vi "swerve_graphing.vi"(10 "wheel offset":dbl format="%_6g", 11 "Pose":dbl[](array[numeric])) -> (2 "Output":cluster{"x out":dbl, "y out":dbl}[](array[cluster]))   [LabVIEW 2020]
uses:
  <vilib>/Analysis/coordinate.llb/2D Cartesian Coordinate Rotation (Scalar).vi
  swerve_globals.vi
  <vilib>/Analysis/NI_AALPro.lvlib
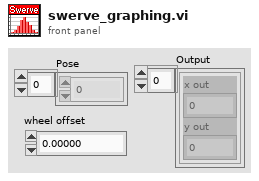
[diagram p1: front panel]
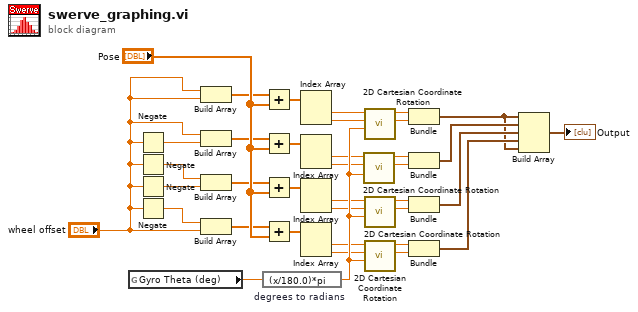
[diagram p0: block diagram]
diagram:
  n1 = global read "swerve_globals.vi" "Gyro Theta (deg)"() -> (w18:dbl)
  n2 = Negate(x="wheel offset") -> (-x=w3:dbl)
  n3 = Negate(x="wheel offset") -> (-x=w1:dbl)
  n4 = Negate(x="wheel offset") -> (-x=w4:dbl)
  n5 = Negate(x="wheel offset") -> (-x=w2:dbl)
  n6 = Build Array("wheel offset", "wheel offset") -> (w24:dbl[])
  n7 = Build Array("wheel offset", w3) -> (w25:dbl[])
  n8 = Build Array(w1, w4) -> (w26:dbl[])
  n9 = Build Array(w2, "wheel offset") -> (w27:dbl[])
  n10 = expression code="(x/180.0)*pi" "degrees to radians"(w18) -> (w23:dbl)
  n11 = Add(x=w24, y="Pose") -> (x+y=w6:dbl[])
  n12 = Add(x=w25, y="Pose") -> (x+y=w7:dbl[])
  n13 = Add(x=w26, y="Pose") -> (x+y=w8:dbl[])
  n14 = Add(x=w27, y="Pose") -> (x+y=w9:dbl[])
  n15 = Index Array(array=w6) -> (element #1=w10:dbl, element #2=w11:dbl)  [unwired: 2 in]
  n16 = Index Array(array=w7) -> (element #1=w12:dbl, element #2=w13:dbl)  [unwired: 2 in]
  n17 = Index Array(array=w8) -> (element #1=w14:dbl, element #2=w15:dbl)  [unwired: 2 in]
  n18 = Index Array(array=w9) -> (element #1=w16:dbl, element #2=w17:dbl)  [unwired: 2 in]
  n19 = call-poly <vilib>:"2D Cartesian Coordinate Rotation.vi"("theta"=w23, "y"=w13, "x"=w12) -> ("y out"=w34:dbl, "x out"=w33:dbl)  [unwired: 6 in, 1 out]
  n20 = call-poly <vilib>:"2D Cartesian Coordinate Rotation.vi"("theta"=w23, "y"=w11, "x"=w10) -> ("y out"=w36:dbl, "x out"=w35:dbl)  [unwired: 6 in, 1 out]
  n21 = call-poly <vilib>:"2D Cartesian Coordinate Rotation.vi"("theta"=w23, "y"=w15, "x"=w14) -> ("y out"=w32:dbl, "x out"=w31:dbl)  [unwired: 6 in, 1 out]
  n22 = call-poly <vilib>:"2D Cartesian Coordinate Rotation.vi"("theta"=w23, "y"=w17, "x"=w16) -> ("y out"=w30:dbl, "x out"=w29:dbl)  [unwired: 6 in, 1 out]
  n23 = Bundle("x out"=w35, "y out"=w36) -> (w19:cluster{"x out":dbl, "y out":dbl})  [unwired: 1 in]
  n24 = Bundle("x out"=w33, "y out"=w34) -> (w20:cluster{"x out":dbl, "y out":dbl})  [unwired: 1 in]
  n25 = Bundle("x out"=w31, "y out"=w32) -> (w21:cluster{"x out":dbl, "y out":dbl})  [unwired: 1 in]
  n26 = Bundle("x out"=w29, "y out"=w30) -> (w22:cluster{"x out":dbl, "y out":dbl})  [unwired: 1 in]
  n27 = Build Array(w19, w20, w21, w22, w19) -> (→"Output":cluster{"x out":dbl, "y out":dbl}[])
